vi "CRYView Out CurLibrary.vi"(8 "DataView Idx":i32, 9 "sData":string="BRIDGE_OUT", 10 "cView":T1, 11 "sAction":string) -> (1 "sData_Out":string="BRIDGE_OUT", 2 "cView_Out":T1)   [LabVIEW 2013]
uses:
  SubVI/CRYData View Global.vi
  CRYView Global.vi
panel:
  out "sName":string
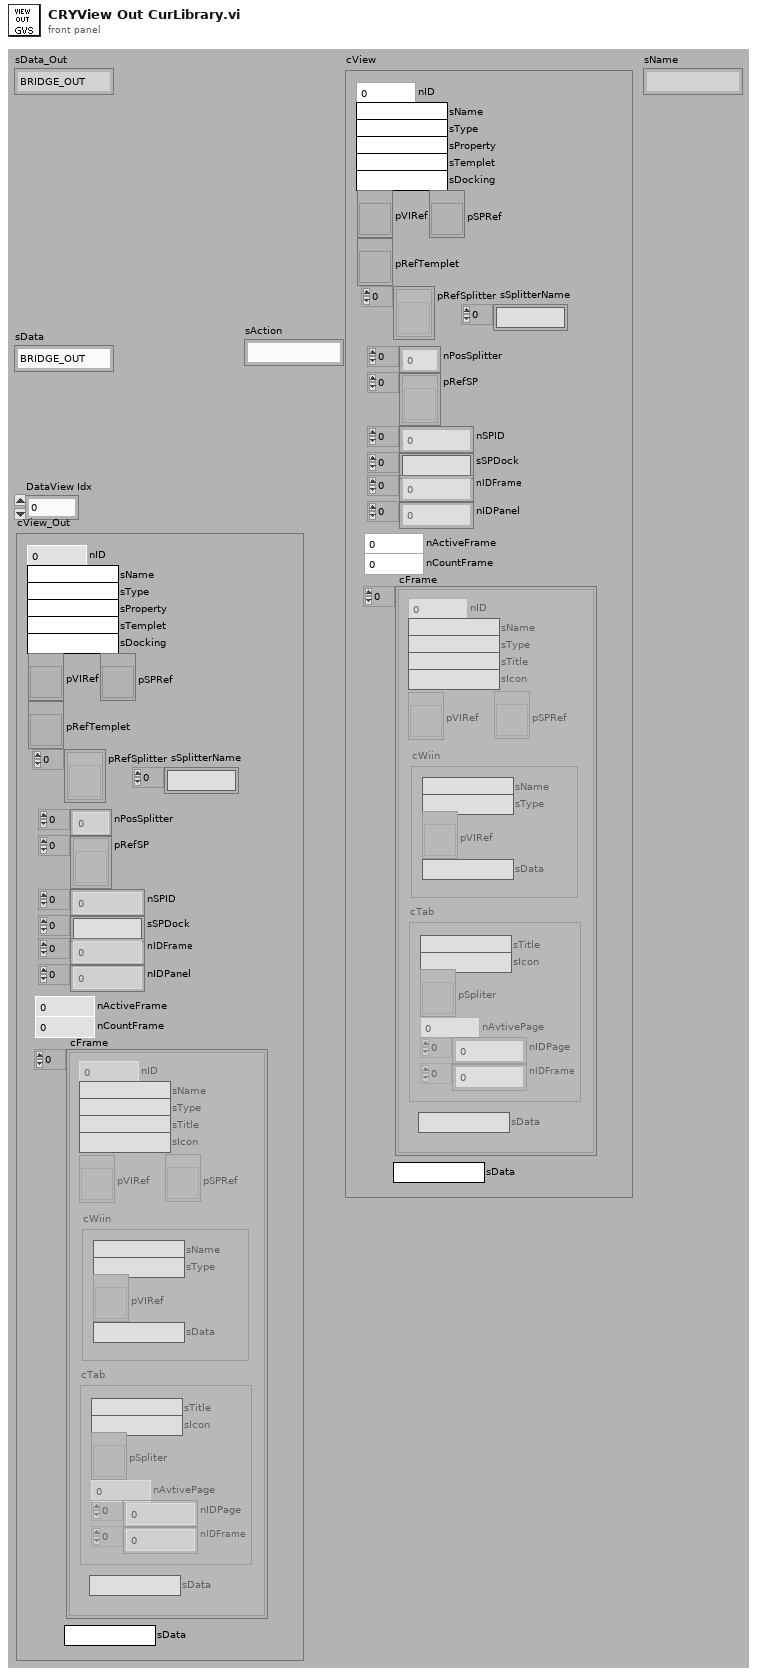
[diagram p1: front panel]
types:
  T1 = cluster{"nID":i32, "sName":string, "sType":string, "sProperty":string, "sTemplet":string, "sDocking":string, "pVIRef":refnum<vi>, "pSPRef":refnum<vi>, "pRefTemplet":refnum<vi>, "pRefSplitter":refnum<vi>[], "nPosSplitter":i32[], "pRefSP":refnum<vi>[], "nSPID":i32[], "sSPDock":string[], "nIDFrame":i32[], "nIDPanel":i32[], "nActiveFrame":i32, "nCountFrame":i32, "cFrame":cluster{"nID":i32, "sName":string, "sType":string, "sTitle":string, "sIcon":string, "pVIRef":refnum<vi>, "pSPRef":refnum<vi>, "cWiin":cluster{"sName":string, "sType":string, "pVIRef":refnum<vi>, "sData":string}, "cTab":cluster{"sTitle":string, "sIcon":string, "pSpliter":refnum<vi>, "nAvtivePage":i32, "nIDPage":i32[], "nIDFrame":i32[]}, "sData":string}[], "sData":string, "sSplitterName":string[]}
  T2 = cluster{"sAction":string, "sData":string, "nData":i32, "pVIRef":refnum<vi>}
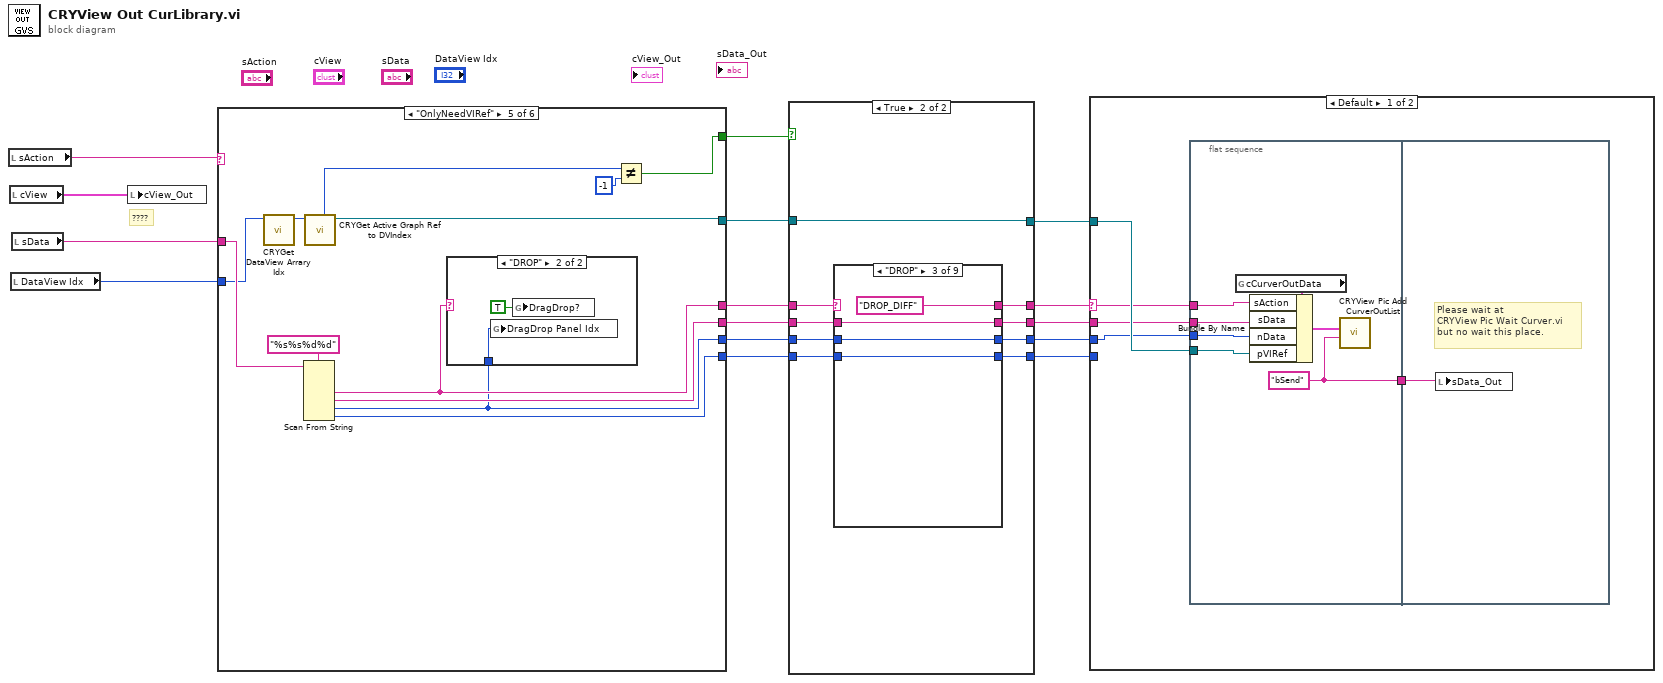
[diagram p0: block diagram]
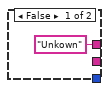
[diagram p3: hidden frame]
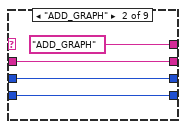
[diagram p5: hidden frame]
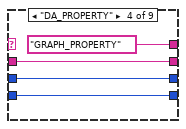
[diagram p6: hidden frame]
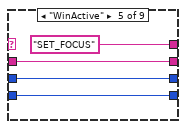
[diagram p7: hidden frame]
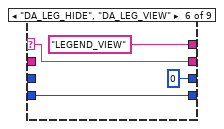
[diagram p8: hidden frame]
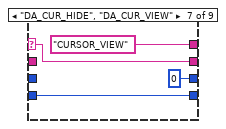
[diagram p9: hidden frame]
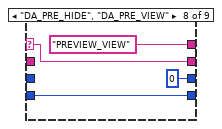
[diagram p10: hidden frame]
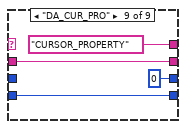
[diagram p11: hidden frame]
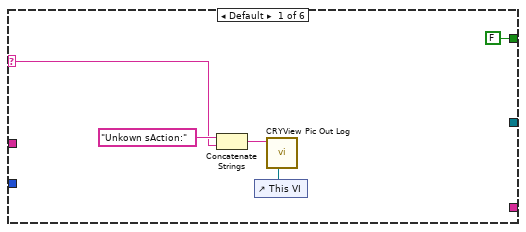
[diagram p12: hidden frame]
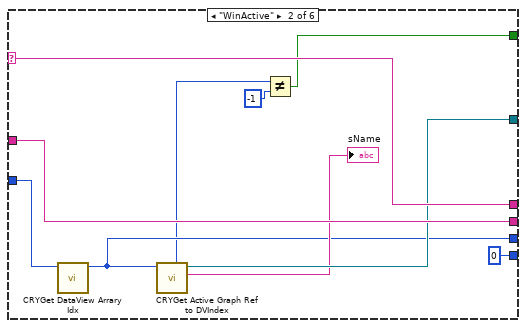
[diagram p13: hidden frame]
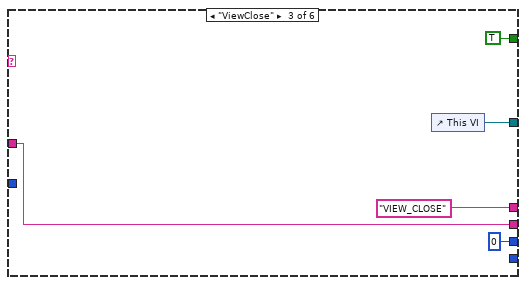
[diagram p14: hidden frame]
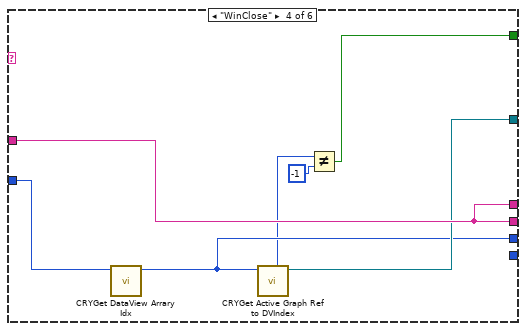
[diagram p15: hidden frame]
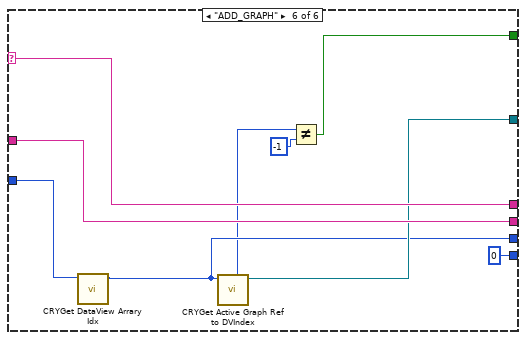
[diagram p17: hidden frame]
diagram:
  # "????"
  n1 = local read "sAction"() -> (w15:string)
  n2 = local read "cView"() -> (w1:T1)
  n3 = local read "DataView Idx"() -> (w8:i32)
  n4 = local read "sData"() -> (w14:string)
  n5 = local write "cView_Out"(w1) -> ()
  n6 = case shown="\"OnlyNeedVIRef\"" w15 {
    selector: w15 -> [w17 w29 _ _ _ w65]
    tunnel: w14 -> [_ w30 w31 w42 w53 w64]
    tunnel: [FALSE w21 TRUE w36 w48 w57] -> w13
    tunnel: [_ w27 w33 w41 w47 w62] -> w7
    tunnel: [_ w29 "VIEW_CLOSE" ("sData") w42 w44 w65] -> w12
    tunnel: [_ w30 w31 w42 w52 w64] -> w11
    tunnel: [_ w24 0 ("nData") w39 w43 w60] -> w10
    tunnel: [_ 0 _ _ w51 0] -> w9
    tunnel: w8 -> [_ w25 _ w40 w50 w61]
    frame Default {
      n7 = Concatenate Strings("Unkown sAction:" ("string"), w17) -> (w20:string)
      n8 = control-ref of="This VI"() -> (w18:refnum<vi>)
      n9 = call "CRYView Pic Out Log.vi"("vi reference"=w18, "sData"=w20) -> ()  [unwired: 10 in]
    }
    frame "WinActive" {
      n10 = call "CRYGet DataView Arrary Idx.vi"("DataView Idx In"=w25) -> ("DataView Arrary Idx out"=w24:i32)  [unwired: 10 in]
      n11 = call "CRYGet Active Graph Ref to DVIndex.vi"("DV Array index"=w24) -> ("sQueueName"=→"sName":string, "Inserted Graph VIRef out"=w27:refnum<vi>, "Graph VIRef Array Index"=w23:i32)  [unwired: 5 in, 3 out]
      n12 = Not Equal?(x=w23, y=-1) -> (x != y?=w21:bool)
    }
    frame "ViewClose" {
      n13 = control-ref of="This VI"() -> (w33:refnum<vi>)
    }
    frame "WinClose" {
      n14 = call "CRYGet DataView Arrary Idx.vi"("DataView Idx In"=w40) -> ("DataView Arrary Idx out"=w39:i32)  [unwired: 10 in]
      n15 = call "CRYGet Active Graph Ref to DVIndex.vi"("DV Array index"=w39) -> ("Inserted Graph VIRef out"=w41:refnum<vi>, "Graph VIRef Array Index"=w37:i32)  [unwired: 5 in, 4 out]
      n16 = Not Equal?(x=w37, y=-1) -> (x != y?=w36:bool)
    }
    frame "OnlyNeedVIRef" {
      n17 = call "CRYGet DataView Arrary Idx.vi"("DataView Idx In"=w50) -> ("DataView Arrary Idx out"=w45:i32)  [unwired: 10 in]
      n18 = Scan From String(format string="%s%s%d%d", input string=w53) -> (output 1=w44:string, output 2=w52:string, output 3=w43:i32, output 4=w51:i32)  [unwired: 2 in, 7 out]
      n19 = call "CRYGet Active Graph Ref to DVIndex.vi"("DV Array index"=w45) -> ("Inserted Graph VIRef out"=w47:refnum<vi>, "Graph VIRef Array Index"=w46:i32)  [unwired: 5 in, 4 out]
      n20 = case shown="\"DROP\"" w44 {
        tunnel: w43 -> [_ w55]
        frame "False", Default {
        }
        frame "DROP" {
          n21 = global write "CRYData View Global.vi" "DragDrop Panel Idx"(w55) -> ()
          n22 = global write "CRYData View Global.vi" "DragDrop?"(TRUE ("DragDrop?")) -> ()
        }
      }
      n23 = Not Equal?(x=w46, y=-1) -> (x != y?=w48:bool)
    }
    frame "ADD_GRAPH" {
      n24 = call "CRYGet DataView Arrary Idx.vi"("DataView Idx In"=w61) -> ("DataView Arrary Idx out"=w60:i32)  [unwired: 10 in]
      n25 = call "CRYGet Active Graph Ref to DVIndex.vi"("DV Array index"=w60) -> ("Inserted Graph VIRef out"=w62:refnum<vi>, "Graph VIRef Array Index"=w58:i32)  [unwired: 5 in, 4 out]
      n26 = Not Equal?(x=w58, y=-1) -> (x != y?=w57:bool)
    }
  }
  n27 = case shown="True" w13 {
    tunnel: w12 -> [_ w75]
    tunnel: w11 -> [_ w74]
    tunnel: w10 -> [_ w73]
    tunnel: w9 -> [_ w72]
    tunnel: ["Unkown" w71] -> w6
    tunnel: [_ w70] -> w5
    tunnel: [_ w69] -> w4
    tunnel: [_ w68] -> w3
    tunnel: [_ w67] -> w2
    tunnel: w7 -> [_ w67]
    frame False {
    }
    frame True {
      n28 = case shown="\"DROP\"" w75 {
        selector: w75 -> [w76 _ _ _ _ w97 w101 w105 _]
        tunnel: w74 -> [w79 w83 w87 w91 w95 _ _ _ w111]
        tunnel: w73 -> [w78 w82 w86 w90 w94 _ _ _ _]
        tunnel: w72 -> [w77 w81 w85 w89 w93 w99 w103 w107 w110]
        tunnel: [w76 "ADD_GRAPH" "DROP_DIFF" "GRAPH_PROPERTY" "SET_FOCUS" "LEGEND_VIEW" "CURSOR_VIEW" "PREVIEW_VIEW" "CURSOR_PROPERTY"] -> w71
        tunnel: [w79 w83 w87 w91 w95 w97 w101 w105 w111] -> w70
        tunnel: [w78 w82 w86 w90 w94 0 ("nData") 0 ("nData") 0 ("nData") 0 ("nData")] -> w69
        tunnel: [w77 w81 w85 w89 w93 w99 w103 w107 w110] -> w68
        frame Default {
        }
        frame "ADD_GRAPH" {
        }
        frame "DROP" {
        }
        frame "DA_PROPERTY" {
        }
        frame "WinActive" {
        }
        frame "DA_LEG_HIDE", "DA_LEG_VIEW" {
        }
        frame "DA_CUR_HIDE", "DA_CUR_VIEW" {
        }
        frame "DA_PRE_HIDE", "DA_PRE_VIEW" {
        }
        frame "DA_CUR_PRO" {
        }
      }
    }
  }
  n29 = case shown="Default" w6 {
    selector: w6 -> [w115 _]
    tunnel: w5 -> [w114 _]
    tunnel: w4 -> [w113 _]
    tunnel: w3 -> [_ _]
    tunnel: w2 -> [w116 _]
    frame Default {
      n30 = flat-sequence {
        tunnel: w116 -> [w122]
        tunnel: w115 -> [w119]
        tunnel: w114 -> [w121]
        tunnel: w113 -> [w120]
        tunnel: [w117] -> w112
        tunnel: w112 -> [w124]
        frame #0 {
          w117 = "bSend" ("Label Name")
          n31 = global read "CRYView Global.vi" "cCurverOutData"() -> (w123:T2)
          n32 = Bundle By Name(cluster=w123, "sAction"=w119, "sData"=w121, "nData"=w120, "pVIRef"=w122) -> (w118:T2)
          n33 = call "CRYView Pic Add CurverOutList.vi"("sName"=w117, "cCurverOutData"=w118) -> ()  [unwired: 10 in]
        }
        frame #1 {
          # "Please wait at \nCRYView Pic Wait Curver.vi\nbut no wait this place."
          n34 = local write "sData_Out"(w124) -> ()
        }
      }
    }
    frame "Unkown" {
      # "Don't know DONG HO sAction"
    }
  }
